vi "Close.vi"(8 "error in (no error)":errorcluster, 11 "Socket.TCP in":refnum<class "Socket.TCP.lvclass">) -> (0 "error out":errorcluster, 3 "Socket.TCP out":refnum<class "Socket.TCP.lvclass">)   [LabVIEW 2014, in "Socket.lvlib" / "Socket.TCP.lvclass"]
doc: "Closes the TCP connection."
uses:
  Socket.TCP.lvclass
  Socket.Base/Socket.Base.lvclass/Socket.Base.ctl
  Socket.TCP.lvclass/Socket.TCP.ctl
  Accessors/Write tcp _refnum.vi
  Accessors/Write listener_refnum.vi
  Socket.Base/Accessors/Write connected.vi
  Socket.Base/Accessors/Read connected.vi
  Accessors/Read tcp _refnum.vi
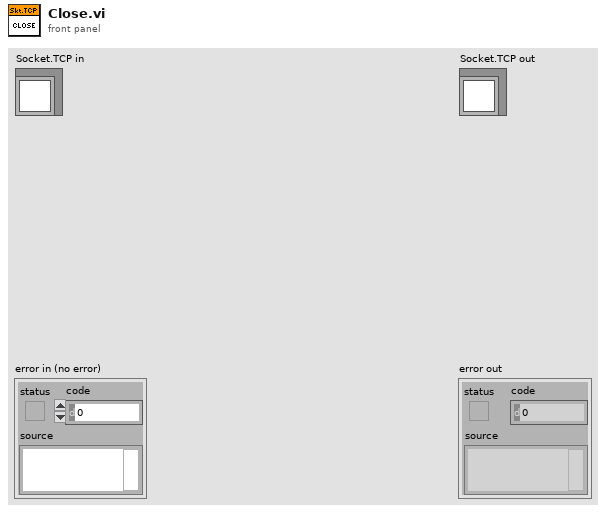
[diagram p1: front panel]
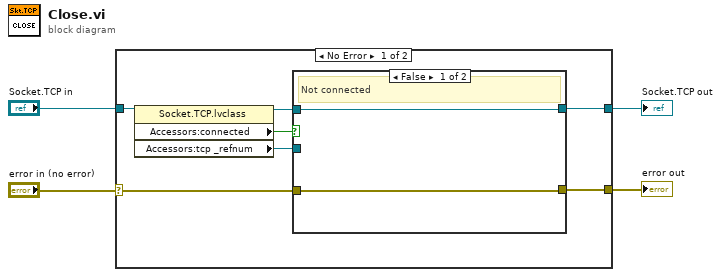
[diagram p0: block diagram]
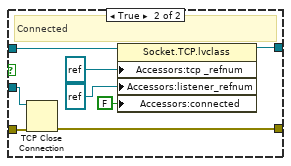
[diagram p2: hidden frame]
diagram:
  n1 = case shown="No Error" "error in (no error)" {
    selector: "error in (no error)" -> [w10 w23]
    tunnel: [w7 w23] -> w3
    tunnel: [w8 w22] -> w1
    tunnel: "Socket.TCP in" -> [w11 w22]
    frame No Error {
      n2 = property class="Socket.TCP.lvclass"(reference=w11) -> (reference out=w9:refnum<class "Socket.TCP.lvclass">, "Accessors:connected"=w5:bool, "Accessors:tcp _refnum"=w6:refnum<k5>)  [unwired: 1 in, 1 out]
      n3 = case shown="False" w5 {
        tunnel: w10 -> [w12 w21]
        tunnel: w9 -> [w13 w20]
        tunnel: [w13 w16] -> w8
        tunnel: [w12 w15] -> w7
        tunnel: w6 -> [_ w14]
        frame False {
          # "Not connected"
        }
        frame True {
          # "Connected"
          n4 = TCP Close Connection(connection ID=w14, error in (no error)=w21) -> (error out=w15:errorcluster)  [unwired: 1 in, 1 out]
          n5 = property class="Socket.TCP.lvclass"(reference=w20, "Accessors:tcp _refnum"=refnum<k5> refnum ("tcp _refnum"), "Accessors:listener_refnum"=refnum<k5> refnum ("listener_refnum"), "Accessors:connected"=FALSE ("connected")) -> (reference out=w16:refnum<class "Socket.TCP.lvclass">)  [unwired: 1 in, 1 out]
        }
      }
    }
    frame Error {
    }
  }
  "error out" <- w3
  "Socket.TCP out" <- w1
